vi "Set trigger.vi"(8 "error in (no error)":errorcluster, 11 "StageSPIM in":refnum<class "StageSPIM.lvclass">) -> (0 "error out":errorcluster, 3 "StageSPIM out":refnum<class "StageSPIM.lvclass">)   [LabVIEW 2012, in "StageSPIM.lvclass"]
uses:
  StageSPIM.lvclass
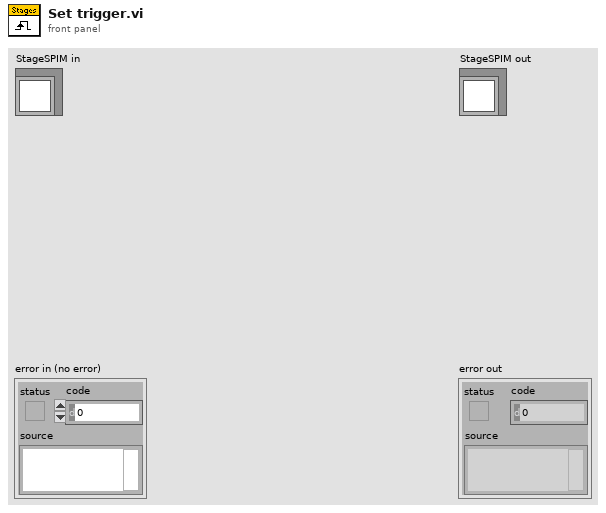
[diagram p1: front panel]
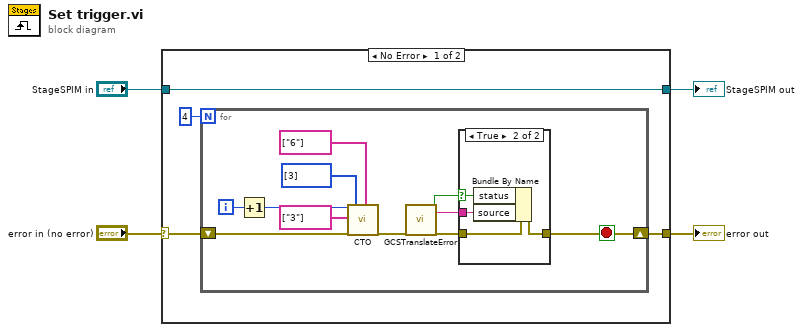
[diagram p0: block diagram]
diagram:
  n1 = case shown="No Error" "error in (no error)" {
    selector: "error in (no error)" -> [w6 w26]
    tunnel: [w5 w26] -> w3
    tunnel: [w8 w25] -> w1
    tunnel: "StageSPIM in" -> [w8 w25]
    frame No Error {
      n2 = for {
        N: 4 -> [_]
        shift-right: [w10] -> w5
        shift-left: w6 -> [w19]
        i -> [w18]
        stop <- w10 stop-if-true
        n3 = Increment(x=w18) -> (x+1=w9:i32)
        n4 = call "CTO.vi"("System no."=w9, "TriggerOut to set"=string[] ["3"], "error in"=w19, "CTO parameter ID"=i32[] [3], "Parameter value"=string[] ["6"]) -> ("error out"=w11:errorcluster)  [unwired: 13 in, 1 out]
        n5 = call "GCSTranslateError.vi"("error in"=w11) -> ("GCS Error?"=w13:bool, "Error Description"=w12:string, "error out"=w14:errorcluster)  [unwired: 16 in]
        n6 = case shown="True" w13 {
          selector: w13 -> [_ w22]
          tunnel: w14 -> [w20 w24]
          tunnel: [w20 w23] -> w10
          tunnel: w12 -> [_ w21]
          frame False {
          }
          frame True {
            n7 = Bundle By Name(cluster=w24, "status"=w22, "source"=w21) -> (w23:errorcluster)
          }
        }
      }
    }
    frame Error {
    }
  }
  "error out" <- w3
  "StageSPIM out" <- w1
